vi "z sample take from loaned.vi"(8 "error in (no error)":errorcluster, 10 "src":cluster{}, 11 "dst":cluster{}) -> (0 "error out":errorcluster, 2 "src out":cluster{}, 3 "dst out":cluster{})   [LabVIEW 2021, in "zenohc.lvlib"]
doc: "void z_sample_take_from_loaned(struct z_owned_sample_t *dst,\n struct z_loaned_sample_t *src);"
uses:
  zenohc.lvlib
  zenohc.dll
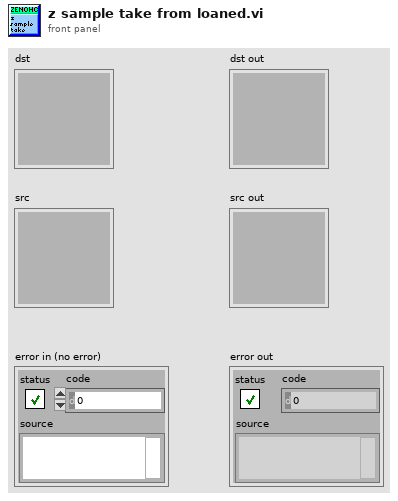
[diagram p1: front panel]
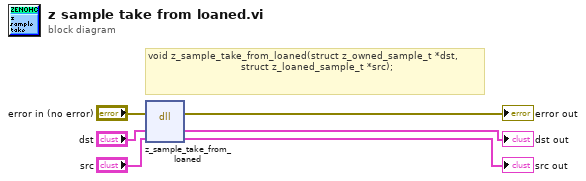
[diagram p0: block diagram]
diagram:
  # "void z_sample_take_from_loaned(struct z_owned_sample_t *dst,\n                               struct z_loaned_sample_t *src);"
  n1 = dll-call lib="D:/dev/zenoh_labview/zenohc/zenohc.*" fn="z_sample_take_from_loaned"(error in="error in (no error)", "dst"="dst", "src"="src") -> (error out=→"error out":errorcluster, "dst"=→"dst out":cluster{}, "src"=→"src out":cluster{})  [unwired: 3 in, 1 out]
